vi "SUB_MAC_CONVERT.vi"(3 "INPUT Encoded MAC":string) -> (1 "ReadableMAC":string)   [LabVIEW 2011]
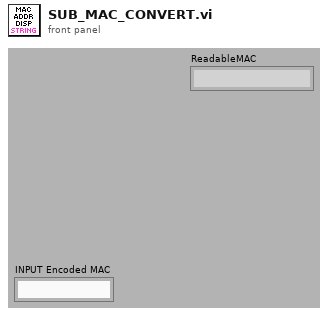
[diagram p1: front panel]
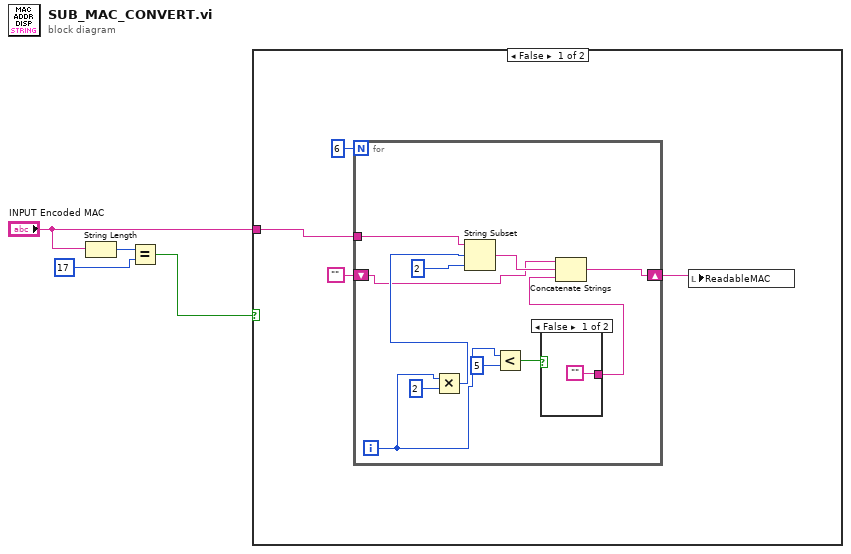
[diagram p0: block diagram]
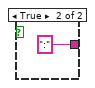
[diagram p2: hidden frame]
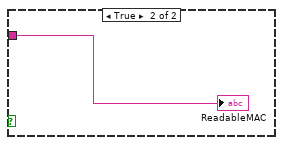
[diagram p3: hidden frame]
diagram:
  n1 = String Length(string="INPUT Encoded MAC") -> (length=w4:i32)
  n2 = Equal?(x=w4, y=17) -> (x = y?=w2:bool)
  n3 = case shown="False" w2 {
    tunnel: "INPUT Encoded MAC" -> [w5 w22]
    frame False {
      n4 = for {
        N: 6 -> [_]
        shift-right: [w15] -> w6
        shift-left: "" -> [w14]
        tunnel: w5 -> [w9]
        i -> [w12]
        n5 = Multiply(x=w12, y=2) -> (x*y=w17:i32)
        n6 = String Subset(string=w9, offset (0)=w17, length (rest)=2 ("length (rest)")) -> (substring=w16:string)
        n7 = Less?(x=w12, y=5) -> (x < y?=w13:bool)
        n8 = case shown="False" w13 {
          tunnel: ["" ":"] -> w10
          frame False {
          }
          frame True {
          }
        }
        n9 = Concatenate Strings(w14, w16, w10) -> (w15:string)
      }
      n10 = local write "ReadableMAC"(w6) -> ()
    }
    frame True {
      "ReadableMAC" <- w22
    }
  }
